vi "writeToXML.vi"(8 "error in (no error)":errorcluster, 10 "ClassLabel":string, 11 "AmLimit in":refnum<class "AmLimit.lvclass">) -> (0 "error out":errorcluster, 2 "XML out":string, 3 "AmLimit out":refnum<class "AmLimit.lvclass">)   [LabVIEW 2014, in "TCSDataDefinitions.lvlib" / "TCSCommand.lvlib" / "AmLimit.lvclass"]
uses:
  AmLimit.lvclass
  AmLimit.lvclass/AmLimit.ctl
  TCSTcsCommand/TCSTcsCommand.lvclass
  <userlib>/Common/XML/XMLGenerator/XMLGenerator.lvclass
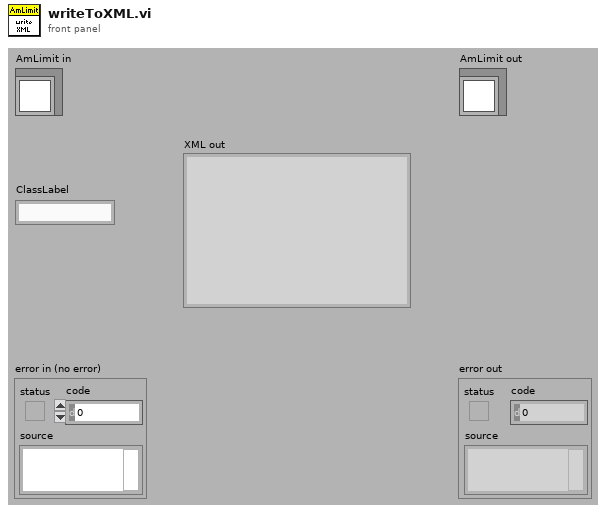
[diagram p1: front panel]
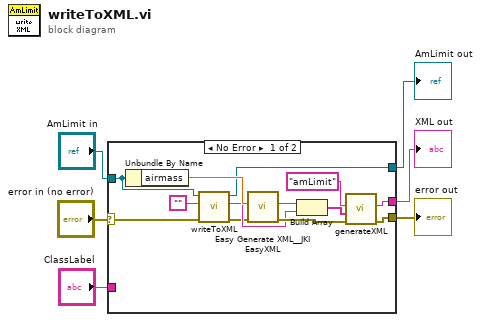
[diagram p0: block diagram]
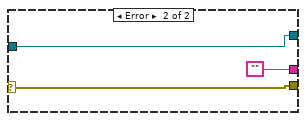
[diagram p2: hidden frame]
diagram:
  n1 = case shown="No Error" "error in (no error)" {
    selector: "error in (no error)" -> [w8 w22]
    tunnel: [w15 w22] -> w5
    tunnel: [w12 w21] -> w3
    tunnel: "AmLimit in" -> [w13 w21]
    tunnel: "ClassLabel" -> [_ _]
    tunnel: [w14 ""] -> w1
    frame No Error {
      n2 = Unbundle By Name(w13) -> ("airmass"=w19:dbl)
      n3 = call-parent "writeToXML.vi"("error in (no error)"=w8, "ClassLabel"="", "TCSTcsCommand in"=w13) -> ("error out"=w7:errorcluster, "XML out"=w10:string, "TCSTcsCommand out"=w12:refnum<class "AmLimit.lvclass">)  [unwired: 6 in]
      n4 = call <vilib>:"Easy Generate XML__JKI EasyXML.vi"("error in (no error)"=w7, "LabVIEW Data"=w19) -> ("error out"=w16:errorcluster, "XML String"=w17:string)  [unwired: 8 in]
      n5 = Build Array(w17, w10) -> (w18:string[])
      n6 = call <userlib>:"generateXML.vi"("error in"=w16, "childrenXML"=w18, "elementName"="amLimit" ("Class Label")) -> ("error out"=w15:errorcluster, "XML out"=w14:string)  [unwired: 6 in, 1 out]
    }
    frame Error {
    }
  }
  "error out" <- w5
  "AmLimit out" <- w3
  "XML out" <- w1
